vi "host.vi"() -> ()   [LabVIEW 2020]
uses:
  <vilib>/rvi/interface/RandomDataEmulation/nirviRandomDataOpen.vi
  <vilib>/rvi/interface/common/niFpgaCacheSessionInfoDynamic.vi
  <vilib>/Utility/error.llb/Error Cluster From Error Code.vi
  <vilib>/rvi/interface/common/niFpgaWaitOnOcc.vi
  <vilib>/rvi/errors/niLvFpgaAdjustHostInterfaceError.vi
  <vilib>/FPGAPlugInAG/Dynamic/niLvFpga_Run_Dynamic.vi
  <vilib>/FPGAPlugInAG/Dynamic/niLvFpga_Close_Dynamic.vi
  <vilib>/rvi/interface/nirviOpenFPGA/nirviOpenFPGA.xnode
  FFT.vi
  <vilib>/rvi/interface/nirviMethod/nirviMethod.xnode
  <vilib>/rvi/interface/nirviCloseFPGA/nirviCloseFPGA.xnode
  <vilib>/rvi/errors/niLvFpgaMergeErrorWithErrorCode.vi
  <vilib>/FPGAPlugInAG/Dynamic/niLvFpga_ReadFifo_Dynamic.vi
  <vilib>/Analysis/NI_AALPro.lvlib
  <vilib>/FPGAPlugInAG/Dynamic/niLvFpga_ConfigureFifo_Dynamic.vi
  <vilib>/FPGAPlugInAG/Dynamic/niLvFpga_StartFifo_Dynamic.vi
  <vilib>/FPGAPlugInAG/Dynamic/niLvFpga_WriteFifo_Dynamic.vi
panel:
  out "truth/restored/final":dbl[][](graph)
  out "final signal trend add":dbl[](graph)
  out "restored   trend add":dbl[](graph)
  out "final signal":fxp<+/-,32,16>[](array[numeric])
  out "final signal":dbl[](graph)
  out "final signal":i32
  out "restored signal":dbl[](graph)
  out "restored signal size":i32
  out "restored signal":fxp<+/-,32,15>[](array[numeric])
  out "phase 2 index":dbl[](graph)
  out "phase 2 size":i32
  out "mag 2 index":dbl[](graph)
  out "mag 2 size":i32
  out "phase 2":fxp<+/-,32,15>[](array[numeric])
  out "mag 2":fxp<+/-,32,15>[](array[numeric])
  out "frequency index":dbl[](graph)
  out "frequency size":i32
  out "freq":fxp<+/-,32,15>[](array[numeric])
  out "magnitude":dbl[](graph)
  out "phase":dbl[](graph)
  out "phase size":i32
  out "mag size":i32
  out "phase":fxp<+/-,32,15>[](array[numeric])
  out "magnitude":fxp<+/-,32,15>[](array[numeric])
  out "Actual Depth":u32
  out "host to target":u32
  out "signal_target_to_host_fixed size(s)":i32
  out "target to host 1":u32
  out "signal target to host":dbl[][](graph)
  out "signal_target_to_host_fixed":fxp<+/-,24,7>[](array[numeric])
  out "Array 2":fxp<+/-,24,7>[](array[numeric])
  out "detrend acc":dbl[](graph)
  out "samples":i32
  out "input signal":T1(graph)
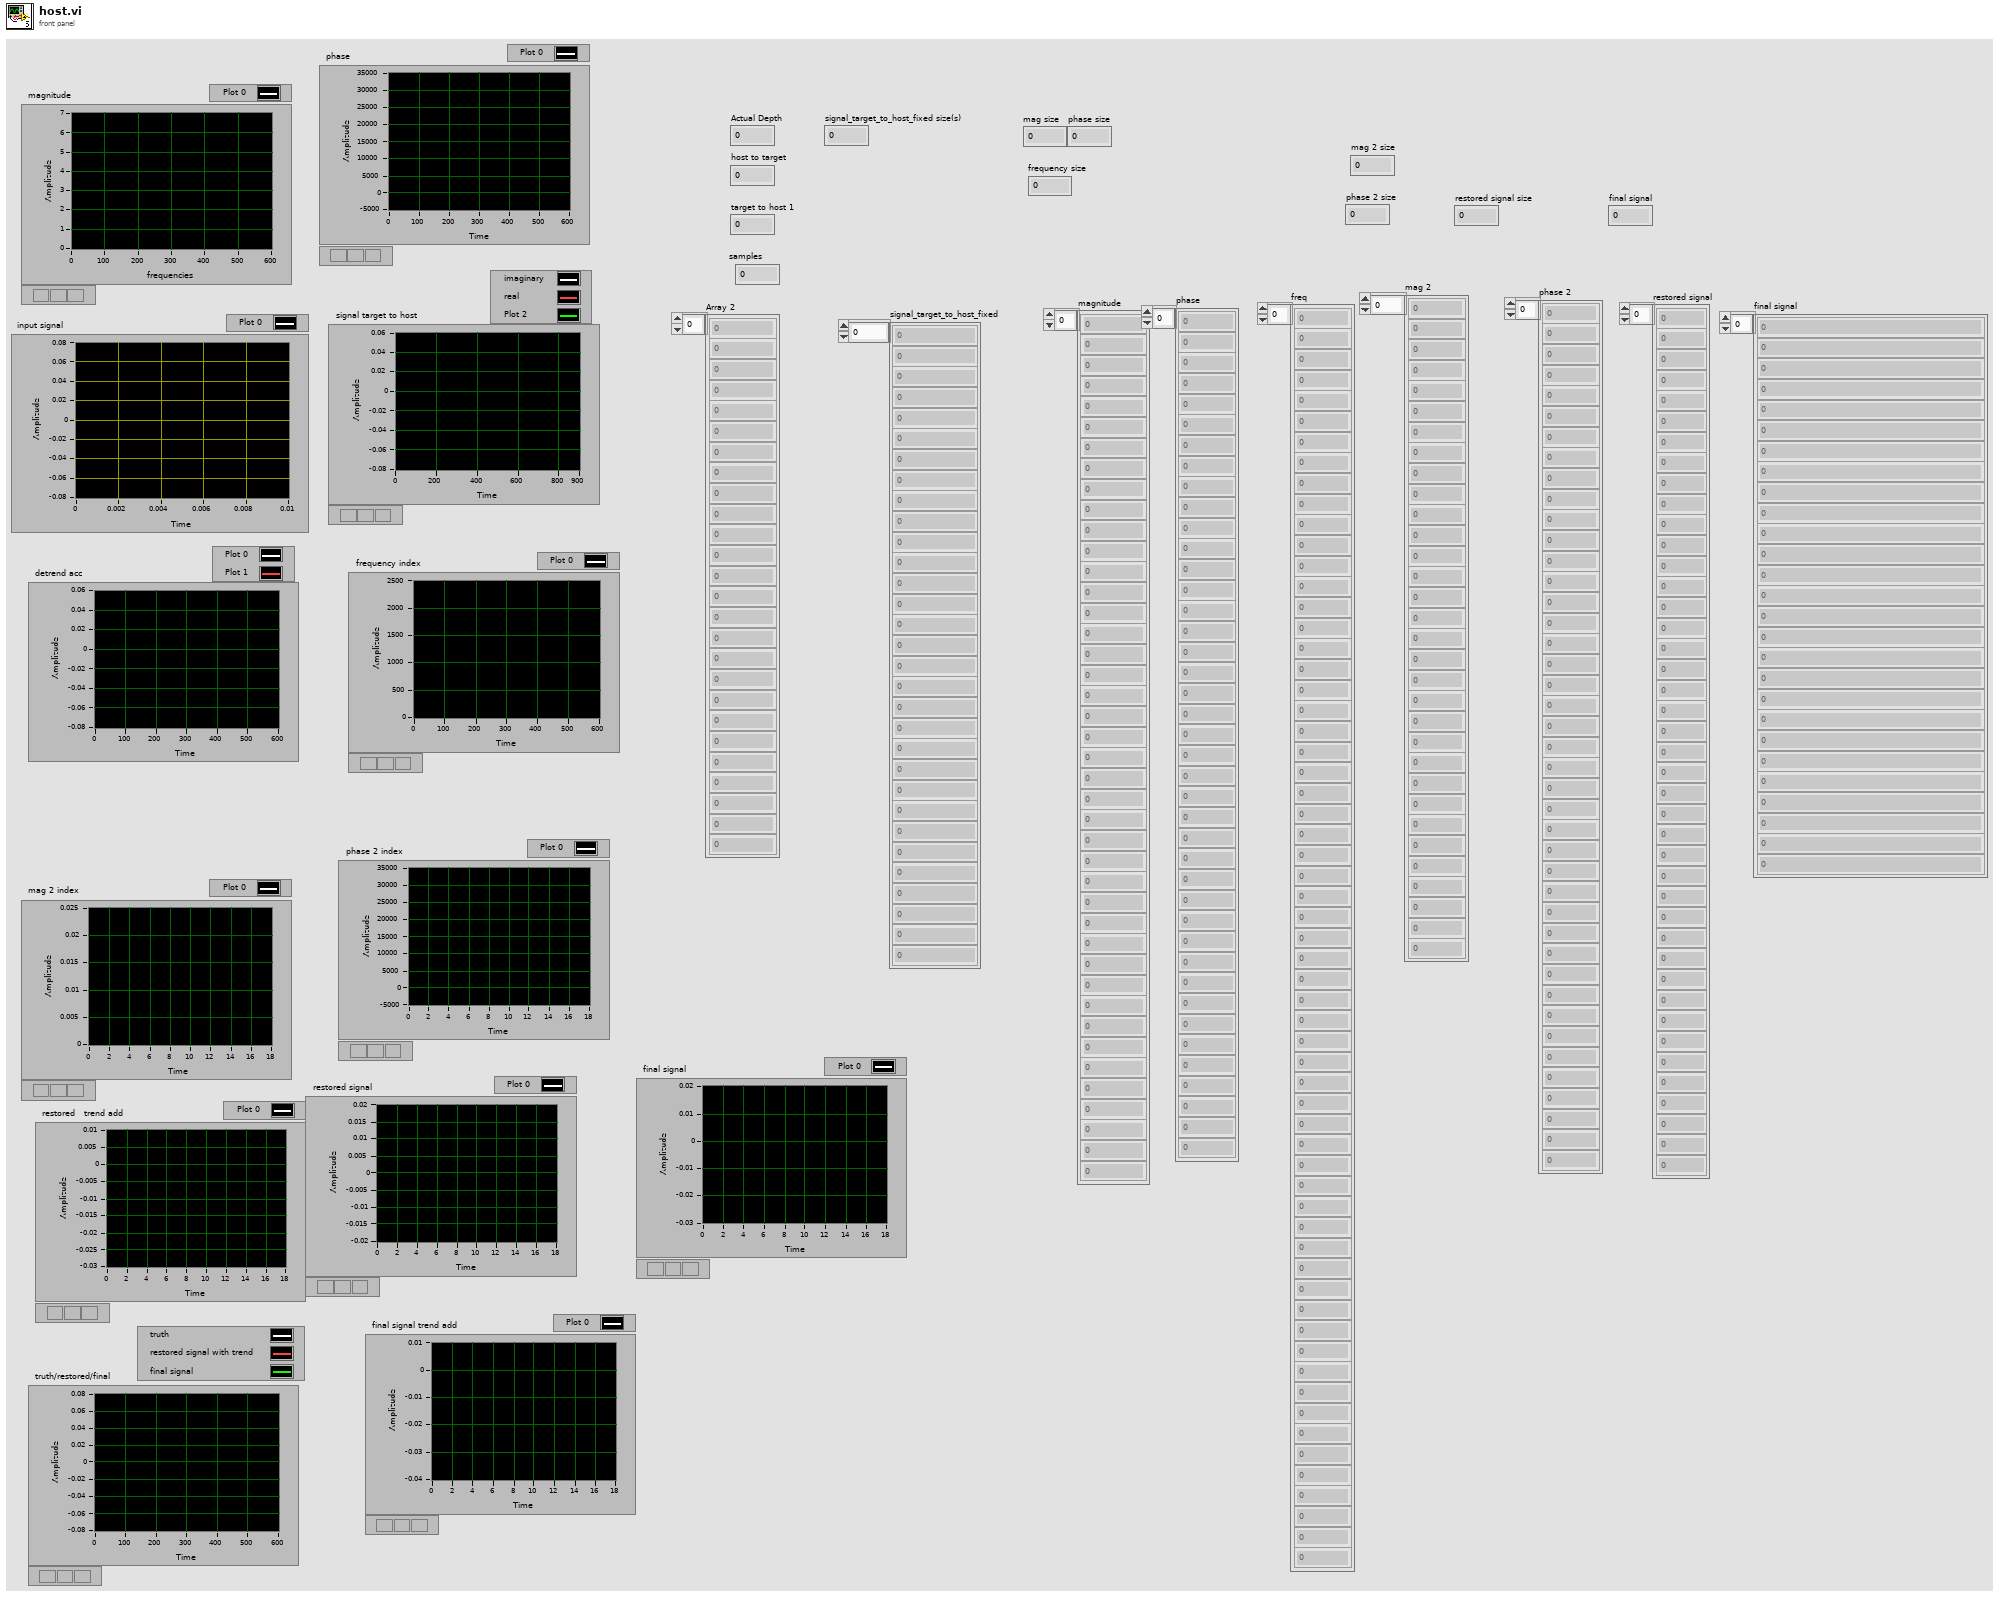
[diagram p1: front panel]
types:
  T1 = cluster{"array type (2D Dbl)":dbl[], "array type (2D Dbl)":dbl[]}
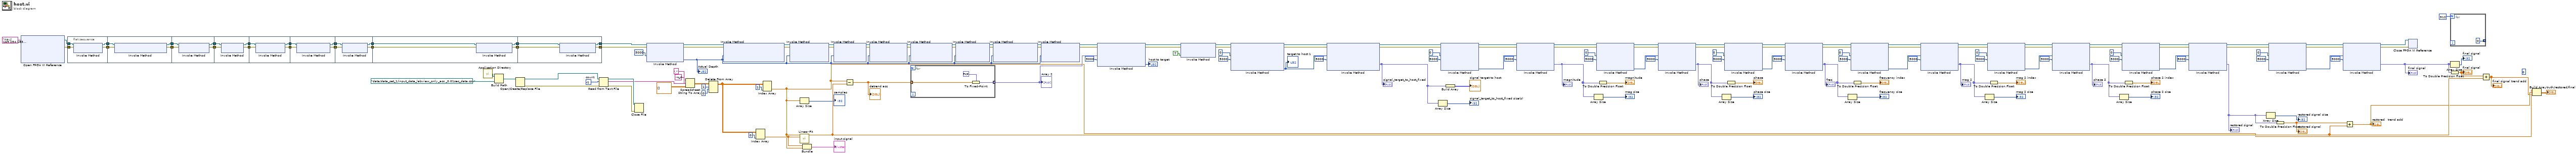
[diagram p0: block diagram]
diagram:
  (unwired) 0 ("index")
  w156 = -1  # count
  n1 = xnode "Open FPGA VI Reference"("resource name"=tag "rio://169.254.183.73/RIO0") -> ("FPGA VI Reference Out"=w126:refnum<k20>, "error out"=w125:errorcluster)  [unwired: 1 in]
  n2 = flat-sequence {
    tunnel: w126 -> [w169]
    tunnel: w125 -> [w168]
    tunnel: [w167] -> w27
    tunnel: [w166] -> w26
    tunnel: w27 -> [w173]
    tunnel: w26 -> [w172]
    tunnel: [w171] -> w25
    tunnel: [w170] -> w24
    tunnel: w25 -> [w177]
    tunnel: w24 -> [w176]
    tunnel: [w175] -> w23
    tunnel: [w174] -> w22
    tunnel: w23 -> [w181]
    tunnel: w22 -> [w180]
    tunnel: [w179] -> w21
    tunnel: [w178] -> w20
    tunnel: w21 -> [w185]
    tunnel: w20 -> [w184]
    tunnel: [w183] -> w19
    tunnel: [w182] -> w18
    tunnel: w19 -> [w189]
    tunnel: w18 -> [w188]
    tunnel: [w187] -> w17
    tunnel: [w186] -> w16
    tunnel: w17 -> [w193]
    tunnel: w16 -> [w192]
    tunnel: [w191] -> w15
    tunnel: [w190] -> w14
    tunnel: w15 -> [w196]
    tunnel: w14 -> [w197]
    tunnel: [w195] -> w13
    tunnel: [w194] -> w12
    tunnel: w13 -> [w201]
    tunnel: w12 -> [w200]
    tunnel: [w199] -> w11
    tunnel: [w198] -> w10
    frame #0 {
      n3 = xnode "Invoke Method"("FPGA VI Reference In"=w169, "error in"=w168) -> ("FPGA VI Reference Out"=w167:refnum<k20>, "error out"=w166:errorcluster)
    }
    frame #1 {
      n4 = xnode "Invoke Method"("FPGA VI Reference In"=w173, "error in"=w172) -> ("FPGA VI Reference Out"=w171:refnum<k20>, "error out"=w170:errorcluster)
    }
    frame #2 {
      n5 = xnode "Invoke Method"("FPGA VI Reference In"=w177, "error in"=w176) -> ("FPGA VI Reference Out"=w175:refnum<k20>, "error out"=w174:errorcluster)
    }
    frame #3 {
      n6 = xnode "Invoke Method"("FPGA VI Reference In"=w181, "error in"=w180) -> ("FPGA VI Reference Out"=w179:refnum<k20>, "error out"=w178:errorcluster)
    }
    frame #4 {
      n7 = xnode "Invoke Method"("FPGA VI Reference In"=w185, "error in"=w184) -> ("FPGA VI Reference Out"=w183:refnum<k20>, "error out"=w182:errorcluster)
    }
    frame #5 {
      n8 = xnode "Invoke Method"("FPGA VI Reference In"=w189, "error in"=w188) -> ("FPGA VI Reference Out"=w187:refnum<k20>, "error out"=w186:errorcluster)
    }
    frame #6 {
      n9 = xnode "Invoke Method"("FPGA VI Reference In"=w193, "error in"=w192) -> ("FPGA VI Reference Out"=w190:refnum<k20>, "error out"=w191:errorcluster)
    }
    frame #7 {
      n10 = xnode "Invoke Method"("FPGA VI Reference In"=w197, "error in"=w196) -> ("FPGA VI Reference Out"=w195:refnum<k20>, "error out"=w194:errorcluster)
    }
    frame #8 {
      n11 = xnode "Invoke Method"("FPGA VI Reference In"=w201, "error in"=w200) -> ("FPGA VI Reference Out"=w199:refnum<k20>, "error out"=w198:errorcluster)
    }
  }
  n12 = call <vilib>:"Application Directory.vi"() -> ("Application Directory"=w160:path)
  n13 = Build Path(base path=w160, name or relative path=path "data/data_set_1/input_data_labview_only_acc _0.01sec_data.csv" ("default name")) -> (appended path=w159:path)
  n14 = Open/Create/Replace File(file path (use dialog)=w159) -> (refnum out=w164:refnum<file>, error out=w165:errorcluster)  [unwired: 5 in, 1 out]
  n15 = Read from Text File(file (use dialog)=w164, count=w156, error in=w165) -> (refnum out=w163:refnum<file>, text=w161:string, error out=w162:errorcluster)  [unwired: 1 in, 1 out]
  n16 = Close File(refnum=w163, error in=w162) -> ()  [unwired: 2 out]
  n17 = xnode "Invoke Method"("FPGA VI Reference In"=w11, "error in"=w10, "Requested Depth"=u32 5000) -> ("FPGA VI Reference Out"=w124:refnum<k20>, "error out"=w123:errorcluster, "Actual Depth"=w32:u32)
  "Actual Depth" <- w32
  n18 = Spreadsheet String To Array(delimiter (Tab)=",", format string="%f", spreadsheet string=w161, array type (2D Dbl)=dbl[][] []) -> (array=w153:dbl[][])
  n19 = Delete From Array(array=w153, length=1, index (row)=0) -> (array with subset deleted=w148:dbl[][])  [unwired: 1 in, 1 out]
  n20 = xnode "Invoke Method"("FPGA VI Reference In"=w124, "error in"=w123, "Requested Depth"=w32) -> ("FPGA VI Reference Out"=w122:refnum<k20>, "error out"=w121:errorcluster)  [unwired: 1 out]
  n21 = Index Array(array=w148, index (col)=0 ("disabled index (col)")) -> (element=w6:dbl[])  [unwired: 1 in]
  n22 = Index Array(array=w148, index (col)=1 ("disabled index (col)")) -> (element=w3:dbl[])  [unwired: 1 in]
  n23 = xnode "Invoke Method"("FPGA VI Reference In"=w122, "error in"=w121, "Requested Depth"=w32) -> ("FPGA VI Reference Out"=w120:refnum<k20>, "error out"=w119:errorcluster)  [unwired: 1 out]
  n24 = Array Size(array=w3) -> (size(s)=→"samples":i32)
  n25 = call <vilib>:"Linear Fit.vi"("Y"=w3, "X"=w6) -> ("Best Linear Fit"=w7:dbl[])  [unwired: 9 in, 4 out]
  n26 = Bundle("array type (2D Dbl)"=w6, "array type (2D Dbl)"=w3) -> (→"input signal":T1)  [unwired: 1 in]
  n27 = xnode "Invoke Method"("FPGA VI Reference In"=w120, "error in"=w119, "Requested Depth"=w32) -> ("FPGA VI Reference Out"=w86:refnum<k20>, "error out"=w85:errorcluster)  [unwired: 1 out]
  n28 = Subtract(x=w3, y=w7) -> (x-y=w140:dbl[])
  "detrend acc" <- w140
  n29 = xnode "Invoke Method"("FPGA VI Reference In"=w86, "error in"=w85, "Requested Depth"=w32) -> ("FPGA VI Reference Out"=w62:refnum<k20>, "error out"=w61:errorcluster)  [unwired: 1 out]
  n30 = xnode "Invoke Method"("FPGA VI Reference In"=w62, "error in"=w61, "Requested Depth"=w32) -> ("FPGA VI Reference Out"=w64:refnum<k20>, "error out"=w63:errorcluster)  [unwired: 1 out]
  n31 = for {
    tunnel: [w203] -> w139 mode=indexing
    tunnel: w140 -> [w202] mode=indexing
    n32 = To Fixed-Point(fixed-point type=fxp<+/-,24,7> 0.0 ("f"), number=w202) -> (fixed-point=w203:fxp<+/-,24,7>)
  }
  "Array 2" <- w139
  n33 = xnode "Invoke Method"("FPGA VI Reference In"=w64, "error in"=w63, "Requested Depth"=w32) -> ("FPGA VI Reference Out"=w47:refnum<k20>, "error out"=w46:errorcluster)  [unwired: 1 out]
  n34 = xnode "Invoke Method"("FPGA VI Reference In"=w47, "error in"=w46, "Requested Depth"=w32) -> ("FPGA VI Reference Out"=w31:refnum<k20>, "error out"=w30:errorcluster)  [unwired: 1 out]
  n35 = xnode "Invoke Method"("FPGA VI Reference In"=w31, "error in"=w30, "Requested Depth"=w32) -> ("FPGA VI Reference Out"=w29:refnum<k20>, "error out"=w28:errorcluster)  [unwired: 1 out]
  n36 = xnode "Invoke Method"("FPGA VI Reference In"=w29, "error in"=w28, "Data"=w139, "Timeout (ms)"=5000) -> ("FPGA VI Reference Out"=w145:refnum<k20>, "error out"=w144:errorcluster, "Empty Elements Remaining"=→"host to target":u32)
  n37 = xnode "Invoke Method"("FPGA VI Reference In"=w145, "error in"=w144, "Wait Until Done (F)"=TRUE) -> ("FPGA VI Reference Out"=w130:refnum<k20>, "error out"=w129:errorcluster)
  n38 = xnode "Invoke Method"("FPGA VI Reference In"=w130, "error in"=w129, "Number of Elements"=u32 0, "Timeout (ms)"=5000) -> ("FPGA VI Reference Out"=w138:refnum<k20>, "error out"=w137:errorcluster, "Elements Remaining"=w136:u32)  [unwired: 1 out]
  "target to host 1" <- w136
  n39 = xnode "Invoke Method"("FPGA VI Reference In"=w138, "error in"=w137, "Number of Elements"=w136, "Timeout (ms)"=5000) -> ("FPGA VI Reference Out"=w101:refnum<k20>, "error out"=w100:errorcluster, "Data"=w132:fxp<+/-,24,7>[])  [unwired: 1 out]
  "signal_target_to_host_fixed" <- w132
  n40 = Array Size(array=w132) -> (size(s)=→"signal_target_to_host_fixed size(s)":i32)
  n41 = xnode "Invoke Method"("FPGA VI Reference In"=w101, "error in"=w100, "Number of Elements"=u32 0, "Timeout (ms)"=5000) -> ("FPGA VI Reference Out"=w115:refnum<k20>, "error out"=w114:errorcluster, "Elements Remaining"=w109:u32)  [unwired: 1 out]
  n42 = Build Array(w132) -> (→"signal target to host":fxp<+/-,24,7>[][])
  n43 = xnode "Invoke Method"("FPGA VI Reference In"=w115, "error in"=w114, "Number of Elements"=w109, "Timeout (ms)"=5000) -> ("FPGA VI Reference Out"=w113:refnum<k20>, "error out"=w112:errorcluster, "Data"=w99:fxp<+/-,32,16>[])  [unwired: 1 out]
  "magnitude" <- w99
  n44 = Array Size(array=w99) -> (size(s)=→"mag size":i32)
  n45 = xnode "Invoke Method"("FPGA VI Reference In"=w113, "error in"=w112, "Number of Elements"=u32 0, "Timeout (ms)"=5000) -> ("FPGA VI Reference Out"=w111:refnum<k20>, "error out"=w110:errorcluster, "Elements Remaining"=w105:u32)  [unwired: 1 out]
  n46 = To Double Precision Float(number=w99) -> (double precision float=→"magnitude":dbl[])
  n47 = xnode "Invoke Method"("FPGA VI Reference In"=w111, "error in"=w110, "Number of Elements"=w105, "Timeout (ms)"=5000) -> ("FPGA VI Reference Out"=w88:refnum<k20>, "error out"=w87:errorcluster, "Data"=w98:fxp<+/-,32,15>[])  [unwired: 1 out]
  "phase" <- w98
  n48 = Array Size(array=w98) -> (size(s)=→"phase size":i32)
  n49 = xnode "Invoke Method"("FPGA VI Reference In"=w88, "error in"=w87, "Number of Elements"=u32 0, "Timeout (ms)"=5000) -> ("FPGA VI Reference Out"=w97:refnum<k20>, "error out"=w96:errorcluster, "Elements Remaining"=w93:u32)  [unwired: 1 out]
  n50 = To Double Precision Float(number=w98) -> (double precision float=→"phase":dbl[])
  n51 = xnode "Invoke Method"("FPGA VI Reference In"=w97, "error in"=w96, "Number of Elements"=w93, "Timeout (ms)"=5000) -> ("FPGA VI Reference Out"=w72:refnum<k20>, "error out"=w71:errorcluster, "Data"=w90:fxp<+/-,32,16>[])  [unwired: 1 out]
  "freq" <- w90
  n52 = Array Size(array=w90) -> (size(s)=→"frequency size":i32)
  n53 = xnode "Invoke Method"("FPGA VI Reference In"=w72, "error in"=w71, "Number of Elements"=u32 0, "Timeout (ms)"=5000) -> ("FPGA VI Reference Out"=w84:refnum<k20>, "error out"=w83:errorcluster, "Elements Remaining"=w80:u32)  [unwired: 1 out]
  n54 = To Double Precision Float(number=w90) -> (double precision float=→"frequency index":dbl[])
  n55 = xnode "Invoke Method"("FPGA VI Reference In"=w84, "error in"=w83, "Number of Elements"=w80, "Timeout (ms)"=5000) -> ("FPGA VI Reference Out"=w70:refnum<k20>, "error out"=w69:errorcluster, "Data"=w66:fxp<+/-,32,16>[])  [unwired: 1 out]
  "mag 2" <- w66
  n56 = Array Size(array=w66) -> (size(s)=→"mag 2 size":i32)
  n57 = xnode "Invoke Method"("FPGA VI Reference In"=w70, "error in"=w69, "Number of Elements"=u32 0, "Timeout (ms)"=5000) -> ("FPGA VI Reference Out"=w78:refnum<k20>, "error out"=w77:errorcluster, "Elements Remaining"=w74:u32)  [unwired: 1 out]
  n58 = To Double Precision Float(number=w66) -> (double precision float=→"mag 2 index":dbl[])
  n59 = xnode "Invoke Method"("FPGA VI Reference In"=w78, "error in"=w77, "Number of Elements"=w74, "Timeout (ms)"=5000) -> ("FPGA VI Reference Out"=w53:refnum<k20>, "error out"=w50:errorcluster, "Data"=w65:fxp<+/-,32,16>[])  [unwired: 1 out]
  "phase 2" <- w65
  n60 = Array Size(array=w65) -> (size(s)=→"phase 2 size":i32)
  n61 = xnode "Invoke Method"("FPGA VI Reference In"=w53, "error in"=w50, "Number of Elements"=u32 0, "Timeout (ms)"=5000) -> ("FPGA VI Reference Out"=w52:refnum<k20>, "error out"=w51:errorcluster, "Elements Remaining"=w55:u32)  [unwired: 1 out]
  n62 = To Double Precision Float(number=w65) -> (double precision float=→"phase 2 index":dbl[])
  n63 = xnode "Invoke Method"("FPGA VI Reference In"=w52, "error in"=w51, "Number of Elements"=w55, "Timeout (ms)"=5000) -> ("FPGA VI Reference Out"=w39:refnum<k20>, "error out"=w38:errorcluster, "Data"=w48:fxp<+/-,64,18>[])  [unwired: 1 out]
  "restored signal" <- w48
  n64 = Array Size(array=w48) -> (size(s)=→"restored signal size":i32)
  n65 = xnode "Invoke Method"("FPGA VI Reference In"=w39, "error in"=w38, "Number of Elements"=u32 0, "Timeout (ms)"=5000) -> ("FPGA VI Reference Out"=w42:refnum<k20>, "error out"=w41:errorcluster, "Elements Remaining"=w35:u32)  [unwired: 1 out]
  n66 = To Double Precision Float(number=w48) -> (double precision float=w9:dbl[])
  "restored signal" <- w9
  n67 = xnode "Invoke Method"("FPGA VI Reference In"=w42, "error in"=w41, "Number of Elements"=w35, "Timeout (ms)"=5000) -> ("FPGA VI Reference Out"=w37:refnum<k20>, "error out"=w36:errorcluster, "Data"=w33:fxp<+/-,32,16>[])  [unwired: 1 out]
  "final signal" <- w33
  n68 = Add(x=w9, y=w7) -> (x+y=w4:dbl[])
  "restored   trend add" <- w4
  n69 = xnode "Close FPGA VI Reference"("FPGA VI Reference In"=w37, "error in"=w36) -> ()  [unwired: 1 out]
  n70 = for {
    N: 512 -> [_]
    tunnel: [0] -> _ mode=indexing
  }
  n71 = Array Size(array=w33) -> (size(s)=→"final signal":i32)
  n72 = To Double Precision Float(number=w33) -> (double precision float=w8:dbl[])
  "final signal" <- w8
  n73 = Add(x=w8, y=w7) -> (x+y=w1:dbl[])
  "final signal trend add" <- w1
  n74 = Build Array(w3, w4, w1) -> (→"truth/restored/final":dbl[][])
